vi "Read System Configuration.vi"(8 "error in":errorcluster, 11 "SystemConfigRepo in":refnum<class "SystemConfigRepo.lvclass">) -> (0 "error out":errorcluster, 2 "System Configuration":refnum<class "PL_System Configuration.lvclass">, 3 "SystemConfigRepo out":refnum<class "SystemConfigRepo.lvclass">)   [LabVIEW 2013, in "PL Framework Configuration Tool.lvlib" / "SystemConfigRepo.lvclass"]
uses:
  SystemConfigRepo.lvclass
  Framework Configuration Classes/system configuration/PL_System Configuration.lvclass
  SystemConfigRepo.lvclass/SystemConfigRepo.ctl
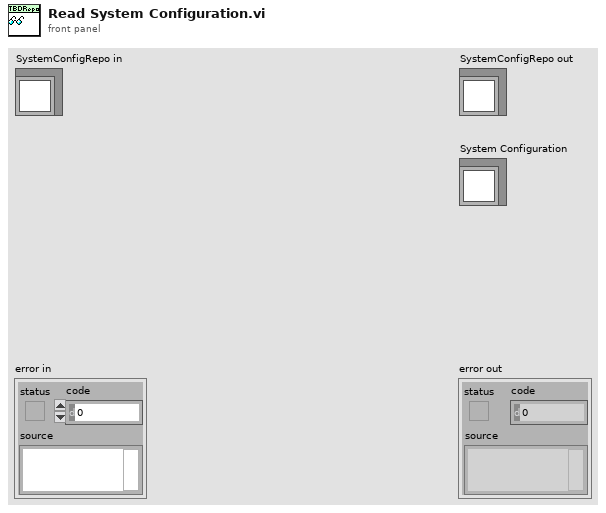
[diagram p1: front panel]
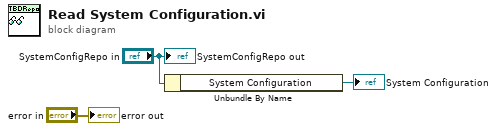
[diagram p0: block diagram]
diagram:
  n1 = Unbundle By Name("SystemConfigRepo in") -> ("System Configuration"=→"System Configuration":refnum<class "PL_System Configuration.lvclass">)
  "error out" <- "error in"
  "SystemConfigRepo out" <- "SystemConfigRepo in"
